vi "generate_random_grid_and_word_list.vi"(11 "Generator Options":T1={"Grid Rows"=300, "Grid Cols"=300, "Word Count"=200, "Max Word Length"=30, "Min Word Length"=5}) -> (2 "Words":string[](array[string]), 3 "Grid":string[][](array[string]))   [LabVIEW 2024, in "Word Search Scorer.lvlib"]
uses:
  Word Search Scorer.lvlib
  Generator Options.ctl
  Letter Index--cluster.ctl
  <vilib>/numeric/Random Number (Range) U64.vi
  <vilib>/numeric/Random Number (Range) I64.vi
  <vilib>/numeric/sub_Random U32.vi
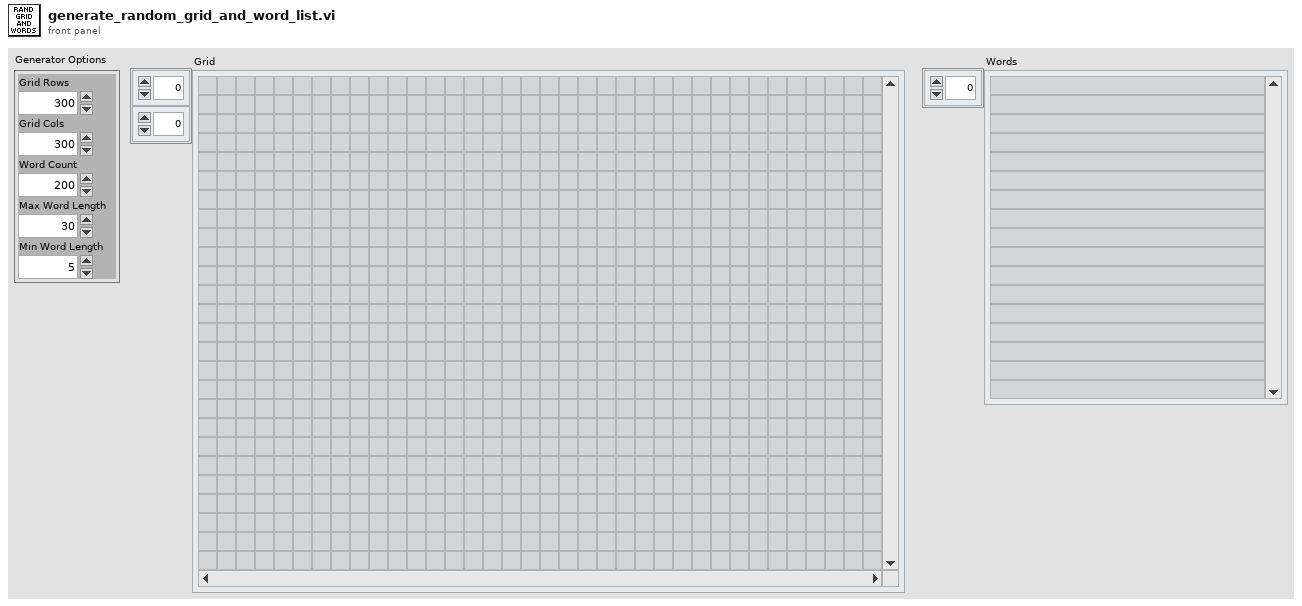
[diagram p1: front panel]
types:
  T1 = typedef "Word Search Scorer.lvlib/Generator Options.ctl" = cluster{"Grid Rows":i32, "Grid Cols":i32, "Word Count":i32, "Max Word Length":u64, "Min Word Length":u64}
  T2 = typedef "Word Search Scorer.lvlib/Letter Index--cluster.ctl" = cluster{"Row":i32, "Column":i32}
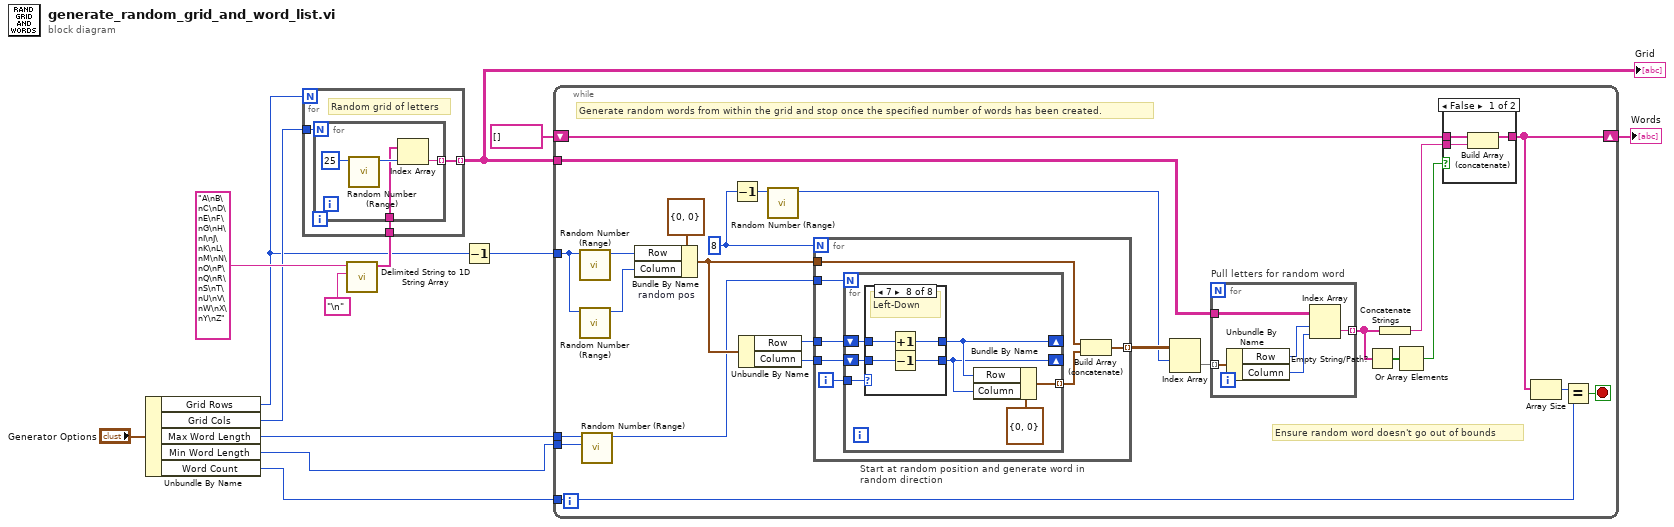
[diagram p0: block diagram]
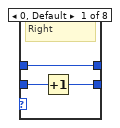
[diagram p3: hidden frame]
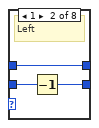
[diagram p4: hidden frame]
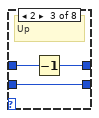
[diagram p5: hidden frame]
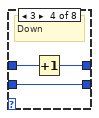
[diagram p6: hidden frame]
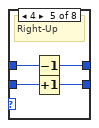
[diagram p7: hidden frame]
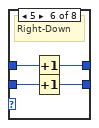
[diagram p8: hidden frame]
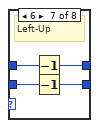
[diagram p9: hidden frame]
diagram:
  n1 = Unbundle By Name("Generator Options") -> ("Grid Rows"=w1:i32, "Grid Cols"=w5:i32, "Max Word Length"=w4:u64, "Min Word Length"=w3:u64, "Word Count"=w2:i32)
  n2 = call <vilib>:"Delimited String to 1D String Array.vi"("delimiter"="\n", "delimited string"="A\nB\nC\nD\nE\nF\nG\nH\nI\nJ\nK\nL\nM\nN\nO\nP\nQ\nR\nS\nT\nU\nV\nW\nX\nY\nZ") -> ("string array"=w11:string[])  [unwired: 9 in]
  n3 = for {
    N: w1 -> [_]
    tunnel: w11 -> [w16]
    tunnel: [w15] -> w10 mode=indexing
    tunnel: w5 -> [w14]
    # "Random grid of letters"
    n4 = for {
      N: w14 -> [_]
      tunnel: w16 -> [w18]
      tunnel: [w17] -> w15 mode=indexing
      n5 = call-poly <vilib>:"Random Number (Range).vi"("upper bound (100)"=u64 25) -> ("number"=w19:u64)  [unwired: 10 in]
      n6 = Index Array(array=w18, index=w19) -> (element=w17:string)
    }
  }
  "Grid" <- w10
  n7 = Decrement(x=w1) -> (x-1=w7:i32)
  n8 = while {
    tunnel: w10 -> [w34]
    shift-right: [w27] -> w8
    shift-left: string[] [] -> [w31]
    tunnel: w7 -> [w24]
    tunnel: w2 -> [w23]
    tunnel: w4 -> [w22]
    tunnel: w3 -> [w21]
    stop <- w26 stop-if-true
    w37 = 8
    # "Generate random words from within the grid and stop once the specified number of words has been created."
    # "Ensure random word doesn't go out of bounds"
    n9 = call-poly <vilib>:"Random Number (Range).vi"("upper bound (100)"=w24) -> ("number"=w42:i64)  [unwired: 10 in]
    n10 = call-poly <vilib>:"Random Number (Range).vi"("upper bound (100)"=w24) -> ("number"=w41:i64)  [unwired: 10 in]
    n11 = call-poly <vilib>:"Random Number (Range).vi"("lower bound (0)"=w21, "upper bound (100)"=w22) -> ("number"=w39:u64)  [unwired: 9 in]
    n12 = Bundle By Name "random pos"(cluster=T2 {"Row"=0, "Column"=0} ("Letter Index"), "Row"=w42, "Column"=w41) -> (w40:T2)
    n13 = Decrement(x=w37) -> (x-1=w38:i32)
    n14 = Unbundle By Name(w40) -> ("Row"=w45:i32, "Column"=w44:i32)
    n15 = call-poly <vilib>:"Random Number (Range).vi"("upper bound (100)"=w38) -> ("number"=w35:u64)  [unwired: 10 in]
    n16 = for "Start at random position and generate word in random direction" {
      N: w37 -> [_]
      tunnel: w39 -> [w61]
      tunnel: w45 -> [w60]
      tunnel: w44 -> [w59]
      tunnel: w40 -> [w56]
      tunnel: [w55] -> w36 mode=indexing
      i -> [w58]
      n17 = for {
        N: w61 -> [_]
        tunnel: w58 -> [w66]
        tunnel: [w64] -> w57 mode=indexing
        shift-right: [w63] -> _
        shift-left: w60 -> [w68]
        shift-right: [w62] -> _
        shift-left: w59 -> [w67]
        n18 = case shown="7" w66 {
          tunnel: w68 -> [w69 w72 w76 w79 w83 w87 w91 w95]
          tunnel: w67 -> [w71 w74 w77 w80 w84 w88 w92 w96]
          tunnel: [w70 w73 w77 w80 w81 w85 w89 w93] -> w62
          tunnel: [w69 w72 w75 w78 w82 w86 w90 w94] -> w63
          frame 0, Default {
            # "Right"
            n19 = Increment(x=w71) -> (x+1=w70:i32)
          }
          frame 1 {
            # "Left"
            n20 = Decrement(x=w74) -> (x-1=w73:i32)
          }
          frame 2 {
            # "Up"
            n21 = Decrement(x=w76) -> (x-1=w75:i32)
          }
          frame 3 {
            # "Down"
            n22 = Increment(x=w79) -> (x+1=w78:i32)
          }
          frame 4 {
            # "Right-Up"
            n23 = Decrement(x=w83) -> (x-1=w82:i32)
            n24 = Increment(x=w84) -> (x+1=w81:i32)
          }
          frame 5 {
            # "Right-Down"
            n25 = Increment(x=w87) -> (x+1=w86:i32)
            n26 = Increment(x=w88) -> (x+1=w85:i32)
          }
          frame 6 {
            # "Left-Up"
            n27 = Decrement(x=w91) -> (x-1=w90:i32)
            n28 = Decrement(x=w92) -> (x-1=w89:i32)
          }
          frame 7 {
            # "Left-Down"
            n29 = Increment(x=w95) -> (x+1=w94:i32)
            n30 = Decrement(x=w96) -> (x-1=w93:i32)
          }
        }
        n31 = Bundle By Name(cluster=T2 {"Row"=0, "Column"=0} ("Letter Index"), "Row"=w63, "Column"=w62) -> (w64:T2)
      }
      n32 = Build Array (concatenate)(w56, w57) -> (w55:T2[])
    }
    n33 = Index Array(array=w36, index (row)=w35) -> (element=w33:T2[])  [unwired: 1 in]
    n34 = for "Pull letters for random word" {
      tunnel: w34 -> [w53]
      tunnel: w33 -> [w54] mode=indexing
      tunnel: [w50] -> w32 mode=indexing
      n35 = Unbundle By Name(w54) -> ("Row"=w52:i32, "Column"=w51:i32)
      n36 = Index Array(array=w53, index (row)=w52, index (col)=w51) -> (element=w50:string)
    }
    n37 = Empty String/Path?(string/path=w32) -> (empty?=w29:bool[])
    n38 = Concatenate Strings(w32) -> (w30:string)
    n39 = Or Array Elements(Boolean array=w29) -> (logical OR=w28:bool)
    n40 = case shown="False" w28 {
      tunnel: w31 -> [w48 w49]
      tunnel: [w47 w49] -> w27
      tunnel: w30 -> [w46 _]
      frame False {
        n41 = Build Array (concatenate)(w48, w46) -> (w47:string[])
      }
      frame True {
      }
    }
    n42 = Array Size(array=w27) -> (size(s)=w25:i32)
    n43 = Equal?(x=w25, y=w23) -> (x = y?=w26:bool)
  }
  "Words" <- w8
